vi "标记周围地块.vi"(2 "索引":i32, 3 "地图":i32[][](array[numeric])) -> (0 "标记个数":i32, 1 "输出地图":i32[][](array[numeric]))   [LabVIEW 2017]
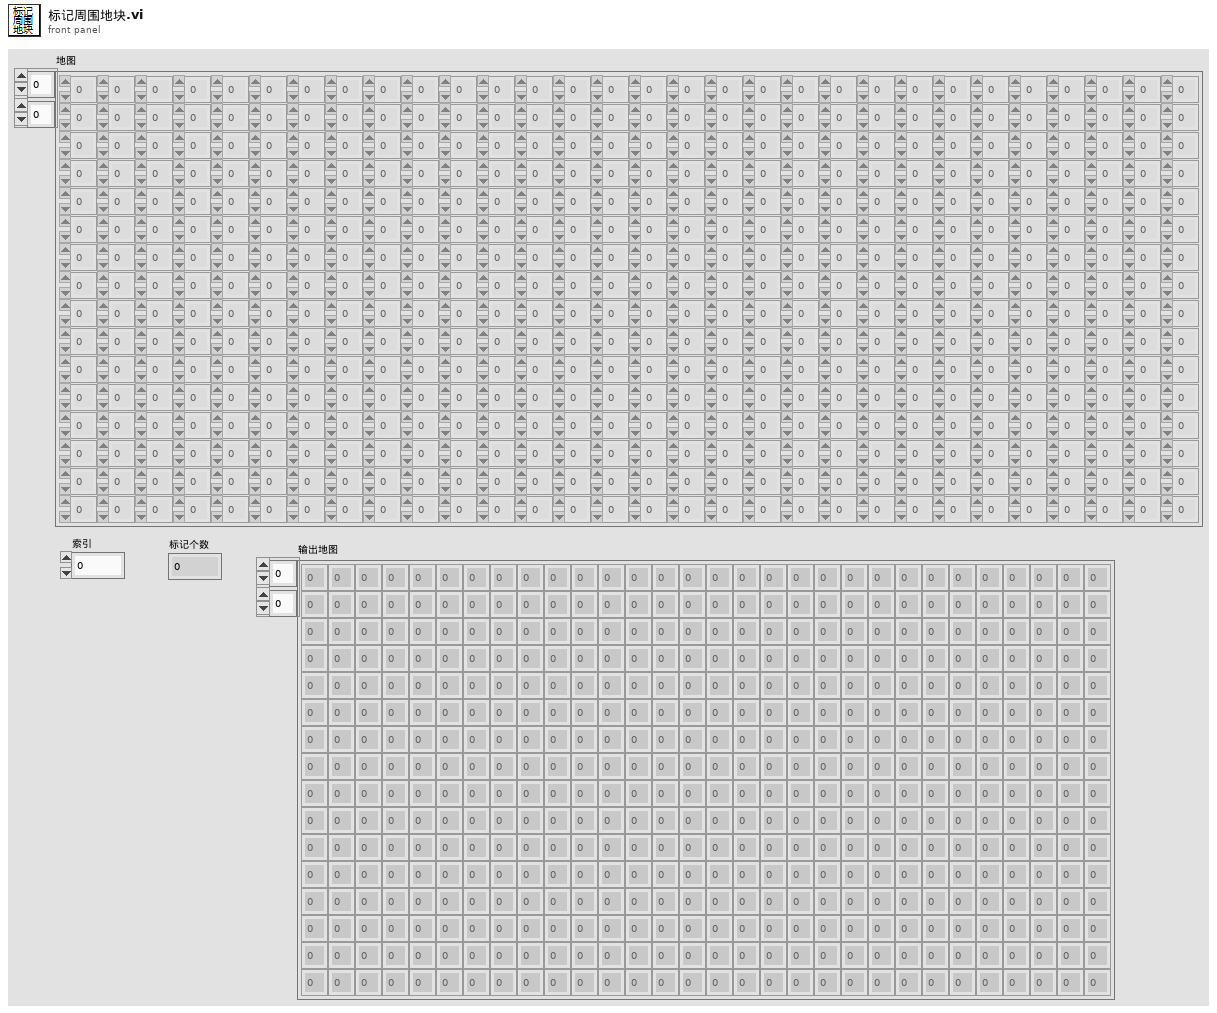
[diagram p1: front panel]
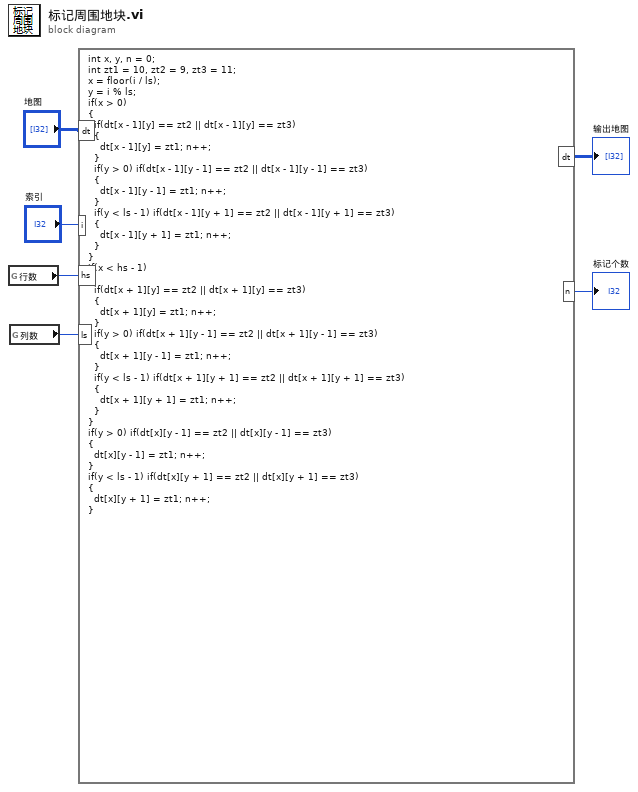
[diagram p0: block diagram]
diagram:
  n1 = global read "全局变量.vi" "行数"() -> (w1:i32)
  n2 = global read "全局变量.vi" "列数"() -> (w2:i32)
  n3 = formula code="int x, y, n = 0;\nint zt1 = 10, zt2 = 9, zt3 = 11;\nx = floor(i / ls);\ny = i % ls;\nif(x > 0)\n{\n  if(dt[x - 1][y] == zt2 || dt[x - 1][y] == zt3)\n  {\n    dt[x - 1][y] = zt1; n++;\n  }\n  if(y > 0) if(dt[x - 1][y - 1] == zt2 || dt[x - 1][y - 1] == zt3)\n  {\n    dt[x - 1][y - 1] = zt1; n++;\n  }\n  if(y < ls - 1) if(dt[x - 1][y + 1] == zt2 || dt[x - 1][y + 1] == zt3)\n  {\n    dt[x - 1][y + 1] = zt1; n++;\n  }\n}\nif(x < hs - 1)\n{\n  if(dt[x + 1][y] == zt2 || dt[x + 1][y] == zt3)\n  {\n    dt[x + 1][y] = zt1; n++;\n  }\n  if(y > 0) if(dt[x + 1][y - 1] == zt2 || dt[x + 1][y - 1] == zt3)\n  {\n    dt[x + 1][y - 1] = zt1; n++;\n  }\n  if(y < ls - 1) if(dt[x + 1][y + 1] == zt2 || dt[x + 1][y + 1] == zt3)\n  {\n    dt[x + 1][y + 1] = zt1; n++;\n  }\n}\nif(y > 0) if(dt[x][y - 1] == zt2 || dt[x][y - 1] == zt3)\n{\n  dt[x][y - 1] = zt1; n++;\n}\nif(y < ls - 1) if(dt[x][y + 1] == zt2 || dt[x][y + 1] == zt3)\n{\n  dt[x][y + 1] = zt1; n++;\n}"("dt"="地图", "i"="索引", "ls"=w2, "hs"=w1) -> ("dt"=→"输出地图":i32[][], "n"=→"标记个数":i32)
